vi "Error.vi"(7 "Error Message":string, 8 "Error In":errorcluster) -> (0 "Error Out":errorcluster)   [LabVIEW 2014]
doc: "Enqueues errors for processing and clears the error flag.\n\nIf there is no error VI does nothing."
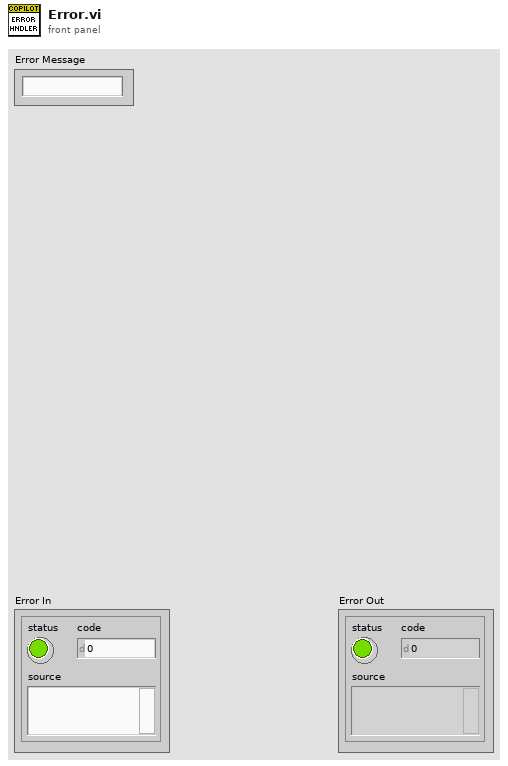
[diagram p1: front panel]
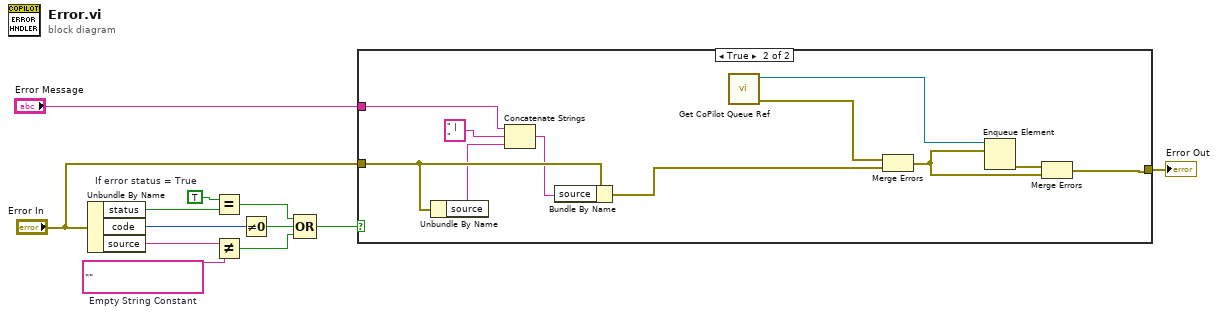
[diagram p0: block diagram]
diagram:
  w8 = ""  # Empty String Constant
  w11 = TRUE  # If error status = True
  n1 = Unbundle By Name("Error In") -> ("status"=w12:bool, "code"=w10:i32, "source"=w9:string)
  n2 = Equal?(x=w11, y=w12) -> (x = y?=w7:bool)
  n3 = Not Equal?(x=w9, y=w8) -> (x != y?=w5:bool)
  n4 = Not Equal To 0?(x=w10) -> (x != 0?=w6:bool)
  n5 = Compound Arithmetic op=OR(w7, w6, w5) -> (w4:bool)
  n6 = case shown="True" w4 {
    tunnel: [w13 w14] -> w2
    tunnel: "Error In" -> [w13 w19]
    tunnel: "Error Message" -> [_ w17]
    frame False {
    }
    frame True {
      n7 = Unbundle By Name(w19) -> ("source"=w16:string)
      n8 = Concatenate Strings(w17, " | " ("string"), w16) -> (w15:string)
      n9 = Bundle By Name(cluster=w19, "source"=w15) -> (w22:errorcluster)
      n10 = call "Get CoPilot Queue Ref.vi"() -> ("Error Out"=w21:errorcluster, "queue out"=w23:refnum<queue>)  [unwired: 10 in]
      n11 = Merge Errors(w21, w22) -> (w20:errorcluster)
      n12 = Enqueue Element(queue=w23, element=w20) -> (error out=w24:errorcluster)  [unwired: 2 in, 2 out]
      n13 = Merge Errors(w24, w20) -> (w14:errorcluster)
    }
  }
  "Error Out" <- w2
